vi "SR400 SetCountParams.vi"(4 "Nb de période":i32=1 min=1 max=2000 step=1, 5 "Counter T Preset (s)":dbl=0.001 min=1e-07 max=90000.0 step=1e-07 format="%#.7g", 6 "error in (no error)":errorcluster, 7 "Dwell time":dbl=6.0 caption="\"Dwell Time\" (s)" min=0.002 max=6.0 step=0.001, 8 "Counter B Preset (s)":dbl=0.001 min=1e-07 max=90000.0 step=1e-07 format="%#.7g", 9 "Mode":u16(ring) items=["A,B for T Preset", "A-B for T Preset", "A+B for T Preset", "A for B preset"], 10 "VISA Port In":refnum<visa-resource-name>="GPIB0::23::INSTR") -> (0 "error out":errorcluster, 3 "VISA Port Out":refnum<visa-resource-name>="GPIB0::23::INSTR")   [LabVIEW 2012]
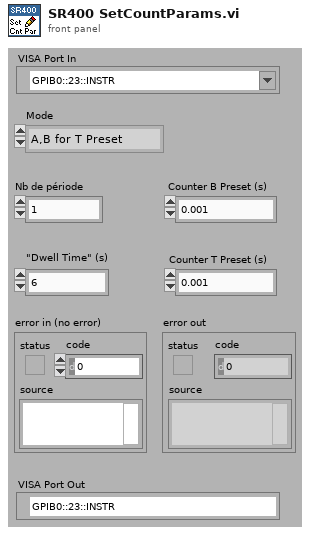
[diagram p1: front panel]
types:
  T1 = enum16{"Lit le Statut", "Configure", "Oper. incomp."}
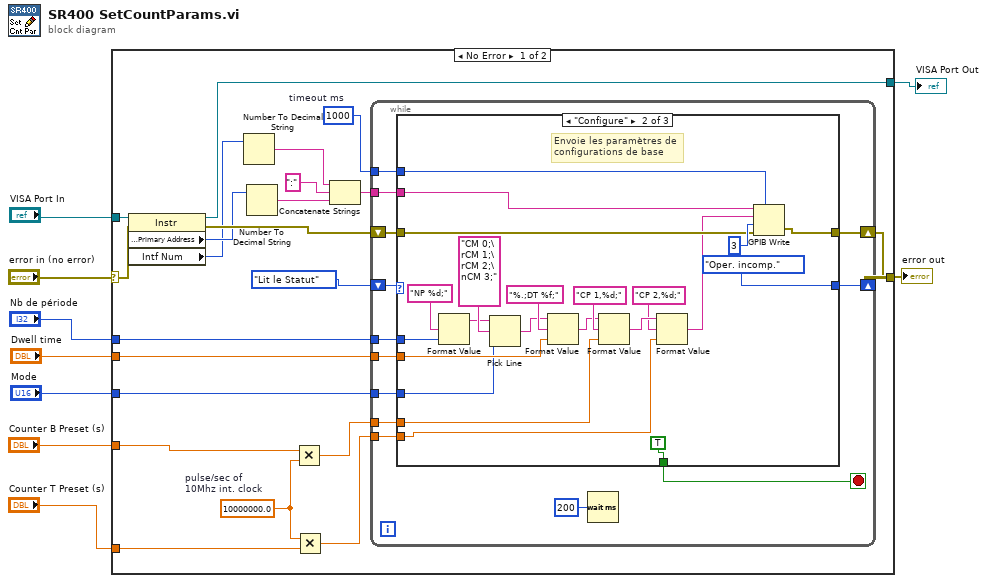
[diagram p0: block diagram]
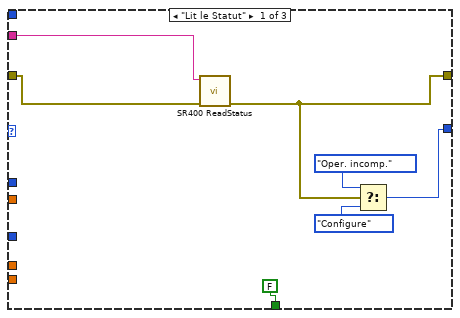
[diagram p2: hidden frame]
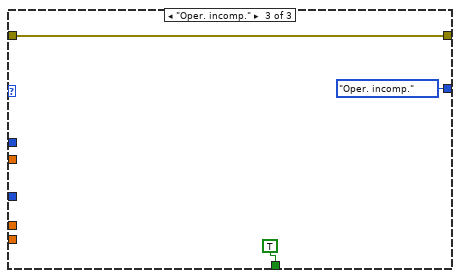
[diagram p3: hidden frame]
diagram:
  n1 = case shown="No Error" "error in (no error)" {
    selector: "error in (no error)" -> [w30 w77]
    tunnel: [w21 w77] -> w8
    tunnel: "VISA Port In" -> [w29 w76]
    tunnel: "Nb de période" -> [w24 _]
    tunnel: "Dwell time" -> [w23 _]
    tunnel: "Mode" -> [w22 _]
    tunnel: "Counter B Preset (s)" -> [w20 _]
    tunnel: "Counter T Preset (s)" -> [w17 _]
    tunnel: [w10 w76] -> w1
    frame No Error {
      w18 = 10000000.0  # pulse/sec of 10Mhz int. clock
      w25 = 1000  # timeout ms
      n2 = property class="Instr"(reference=w29, error in=w30) -> (reference out=w10:refnum<visa-resource-name>, error out=w28:errorcluster, "GPIB Settings:Primary Address"=w26:u16, "Intf Num"=w15:u16)
      n3 = Number To Decimal String(number=w15) -> (decimal integer string=w12:string)  [unwired: 1 in]
      n4 = Number To Decimal String(number=w26) -> (decimal integer string=w13:string)  [unwired: 1 in]
      n5 = Multiply(x=w20, y=w18) -> (x*y=w19:dbl)
      n6 = Multiply(x=w18, y=w17) -> (x*y=w16:dbl)
      n7 = Concatenate Strings(w12, ":" ("string"), w13) -> (w14:string)
      n8 = while {
        shift-right: [w35] -> _
        shift-left: T1."Lit le Statut" -> [w43]
        tunnel: w14 -> [w41]
        shift-right: [w40] -> w21
        shift-left: w28 -> [w42]
        tunnel: w25 -> [w39]
        tunnel: w24 -> [w38]
        tunnel: w23 -> [w37]
        tunnel: w22 -> [w34]
        tunnel: w19 -> [w33]
        tunnel: w16 -> [w31]
        stop <- w36 stop-if-true
        n9 = case shown="\"Configure\"" w43 {
          tunnel: w42 -> [w49 w71 w75]
          tunnel: w41 -> [w48 w70 _]
          tunnel: [w44 w51 w75] -> w40
          tunnel: w39 -> [_ w69 _]
          tunnel: w38 -> [_ w67 _]
          tunnel: w37 -> [_ w65 _]
          tunnel: [FALSE ("Configuration\neffectuée") TRUE ("Configuration\neffectuée") TRUE ("Configuration\neffectuée")] -> w36
          tunnel: [w45 T1."Oper. incomp." T1."Oper. incomp."] -> w35
          tunnel: w34 -> [_ w60 _]
          tunnel: w33 -> [_ w59 _]
          tunnel: w31 -> [_ w53 _]
          frame "Lit le Statut" {
            n10 = call <userlib>:"SR400 ReadStatus.vi"("error in"=w49, "Address string"=w48) -> ("Error Out"=w44:errorcluster)  [unwired: 6 in, 1 out]
            n11 = Select(t=T1."Oper. incomp.", s=w44, f=T1."Configure") -> (s? t:f=w45:T1)
          }
          frame "Configure" {
            # "Envoie les paramètres de configurations de base"
            n12 = Format Value(format string="NP %d;", value (0)=w67) -> (output string=w62:string)  [unwired: 1 in]
            n13 = Pick Line(string ("")=w62, multi-line string="CM 0;\rCM 1;\rCM 2;\nCM 3;", line index=w60) -> (output string=w61:string)
            n14 = Format Value(string ("")=w61, format string="%.;DT %f;", value (0)=w65) -> (output string=w57:string)
            n15 = Format Value(string ("")=w57, format string="CP 1,%d;", value (0)=w59) -> (output string=w55:string)
            n16 = Format Value(string ("")=w55, format string="CP 2,%d;", value (0)=w53) -> (output string=w52:string)
            n17 = GPIB Write(0:w70, 1:w52, 2:i16 3 ("mode (0)"), 3:w71, 4:w69) -> (6:w51:errorcluster)  [unwired: 1 out]
          }
          frame "Oper. incomp." {
          }
        }
        n18 = Wait (ms)(milliseconds to wait=u32 200) -> ()  [unwired: 1 out]
      }
    }
    frame Error {
    }
  }
  "error out" <- w8
  "VISA Port Out" <- w1
